vi "Open Send Dialog.vi"   [LabVIEW 2011, in "CAN FD.lvlib"]
uses:
  CAN FD.lvlib
  Send Dialog.vi
types:
  T1 = enum32{"Bad", "Idle", "Run top level", "Running"}
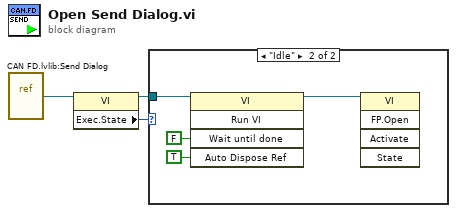
[diagram p0: block diagram]
diagram:
  n1 = vi-ref "CAN FD.lvlib:Send Dialog.vi"() -> (w3:refnum<vi>)
  n2 = property class="VI"(reference=w3) -> (reference out=w1:refnum<vi>, "Exec.State"=w2:T1)  [unwired: 1 in, 1 out]
  n3 = case shown="\"Idle\"" w2 {
    tunnel: w1 -> [_ w7]
    frame "Bad", Default {
    }
    frame "Idle" {
      n4 = invoke class="VI" method="Run VI"(reference=w7, "Wait until done"=FALSE ("结束前等待"), "Auto Dispose Ref"=TRUE ("自动销毁引用")) -> (reference out=w4:refnum<vi>)  [unwired: 2 in, 4 out]
      n5 = invoke class="VI" method="FP.Open"(reference=w4) -> ()  [unwired: 4 in, 5 out]
    }
  }
